vi "Cascade MEMS Only Reliability Gen 0 Header Ver1.0.vi"(8 "Error In":errorcluster, 11 "Measurement Header":string[](array[string])=["CMin_0(fF)", "C1_Max(fF)", "CMin_1(fF)", "C3_Max(fF)", "CMin_2(fF)", "C4_Max(fF)", "CMin_3(fF)", "C2_Max(fF)", "CMin_4(fF)", "C5_Max(fF)", "CMin_5(fF)", "C6_Max(fF)", "CMin_6(fF)", "C145_Max(fF)", "CMin_7(fF)", "C236_Max(fF)", "CMin_8(fF)", "Delta_C1(fF)", "Delta_C3(fF)", "Delta_C4(fF)", "Delta_C2(fF)", "Delta_C5(fF)", "Delta_C6(fF)", "%Delta_C1", "%Delta_C3", "%Delta_C4", "%Delta_C2", "%Delta_C5", "%Delta_C6"]) -> (0 "Error Out":errorcluster, 3 "Name Calculated Header":string[](array[string]))   [LabVIEW 2017]
panel:
  in  "Measurement VPI Header":string[](array[string])=["VPI_Voltage(V)", "VPI_C1_Max(fF)", "VPI_C1_Min(fF)", "VPI_C3_Max(fF)", "VPI_C3_Min(fF)", "VPI_C4_Max(fF)", "VPI_C4_Min(fF)", "VPI_C2_Max(fF)", "VPI_C2_Min(fF)", "VPI_C5_Max(fF)", "VPI_C5_Min(fF)", "VPI_C6_Max(fF)", "VPI_C6_Min(fF)", "VPI_DCAP_C1(fF)", "VPI_DCAP_C3(fF)", "VPI_DCAP_C4(fF)", "VPI_DCAP_C2(fF)", "VPI_DCAP_C5(fF)", "VPI_DCAP_C6(fF)"]
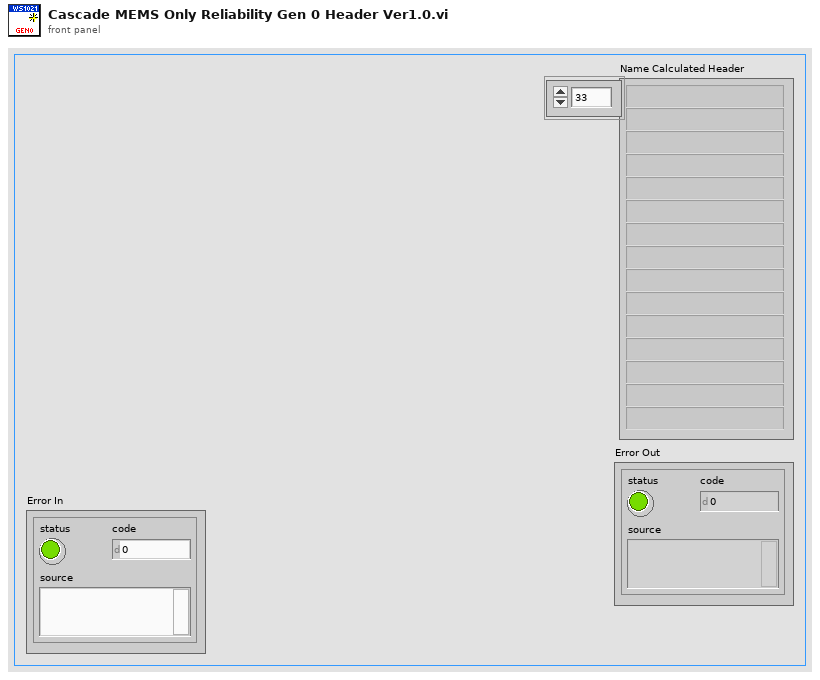
[diagram p1: front panel]
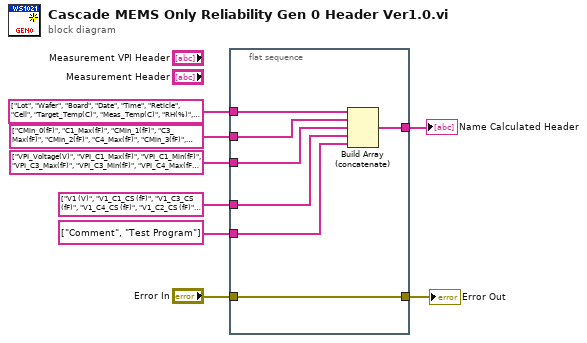
[diagram p0: block diagram]
diagram:
  n1 = flat-sequence {
    tunnel: "Error In" -> [w15]
    tunnel: [w15] -> w8
    tunnel: string[] ["Lot", "Wafer", "Board", "Date", "Time", "Reticle", "Cell", "Target_Temp(C)", "Meas_Temp(C)", "RH(%)", "Freq (KHz)", "Stress_V(V)", "Stress_Beams", "Duty Cycle(%)", "Stress(Min/Num)"] -> [w14]
    tunnel: string[] ["CMin_0(fF)", "C1_Max(fF)", "CMin_1(fF)", "C3_Max(fF)", "CMin_2(fF)", "C4_Max(fF)", "CMin_3(fF)", "C2_Max(fF)", "CMin_4(fF)", "C5_Max(fF)", "CMin_5(fF)", "C6_Max(fF)", "CMin_6(fF)", "C145_Max(fF)", "CMin_7(fF)", "C236_Max(fF)", "CMin_8(fF)", "Delta_C1(fF)", "Delta_C3(fF)", "Delta_C4(fF)", "Delta_C2(fF)", "Delta_C5(fF)", "Delta_C6(fF)", "Delta_C145(fF)", "Delta_C236(fF)", "%Delta_C1", "%Delta_C3", "%Delta_C4", "%Delta_C2", "%Delta_C5", "%Delta_C6"] ("Measurement Header") -> [w13]
    tunnel: [w12] -> w6
    tunnel: string[] ["VPI_Voltage(V)", "VPI_C1_Max(fF)", "VPI_C1_Min(fF)", "VPI_C3_Max(fF)", "VPI_C3_Min(fF)", "VPI_C4_Max(fF)", "VPI_C4_Min(fF)", "VPI_C2_Max(fF)", "VPI_C2_Min(fF)", "VPI_C5_Max(fF)", "VPI_C5_Min(fF)", "VPI_C6_Max(fF)", "VPI_C6_Min(fF)", "VPI_DCAP_C1(fF)", "VPI_DCAP_C3(fF)", "VPI_DCAP_C4(fF)", "VPI_DCAP_C2(fF)", "VPI_DCAP_C5(fF)", "VPI_DCAP_C6(fF)", "VPI_%Delta_C1", "VPI_%Delta_C3", "VPI_%Delta_C4", "VPI_%Delta_C2", "VPI_%Delta_C5", "VPI_%Delta_C6"] ("Measurement VPI Header") -> [w11]
    tunnel: string[] ["Comment", "Test Program"] -> [w9]
    tunnel: string[] ["V1 (V)", "V1_C1_CS (fF)", "V1_C3_CS (fF)", "V1_C4_CS (fF)", "V1_C2_CS (fF)", "V1_C5_CS (fF)", "V1_C6_CS (fF)", "V2 (V)", "V2_C1_CS (fF)", "V2_C3_CS (fF)", "V2_C4_CS (fF)", "V2_C2_CS (fF)", "V2_C5_CS (fF)", "V2_C6_CS (fF)", "V3 (V)", "V3_C1_CS (fF)", "V3_C3_CS (fF)", "V3_C4_CS (fF)", "V3_C2_CS (fF)", "V3_C5_CS (fF)", "V3_C6_CS (fF)", "VCmin_C1(V)", "VCmin_C3(V)", "VCmin_C4(V)", "VCmin_C2(V)", "VCmin_C5(V)", "VCmin_C6(V)"] -> [w10]
    frame #0 {
      n2 = Build Array (concatenate)(w14, w13, w11, w10, w9) -> (w12:string[])
    }
  }
  "Name Calculated Header" <- w6
  "Error Out" <- w8
